vi "User32dllAPI.EnumWindows.vi"(8 "error in (no error)":errorcluster, 10 "Pattern":string, 11 "hWnd in (NULL)":i32) -> (0 "error out":errorcluster, 1 "ClassName":string[](array[string]), 2 "WindowName":string[](array[string]), 3 "hWnd out":i32)   [LabVIEW 2016]
uses:
  <vilib>/Utility/importsl/GetValueByPointer/datatype.ctl
  <vilib>/Utility/importsl/GetValueByPointer/GetValueByPointer.xnode
  User32WinApi.dll
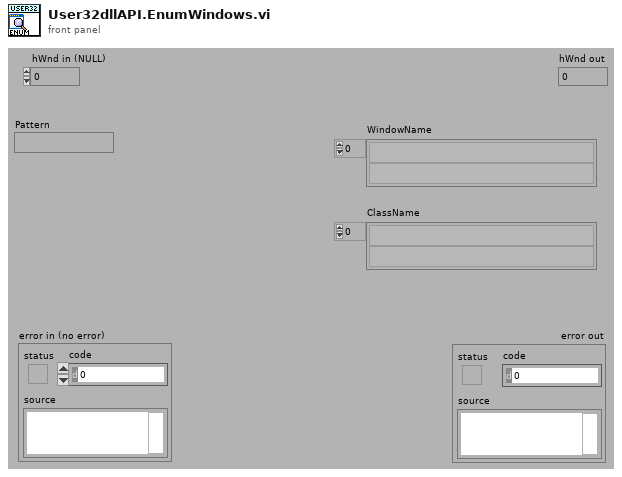
[diagram p1: front panel]
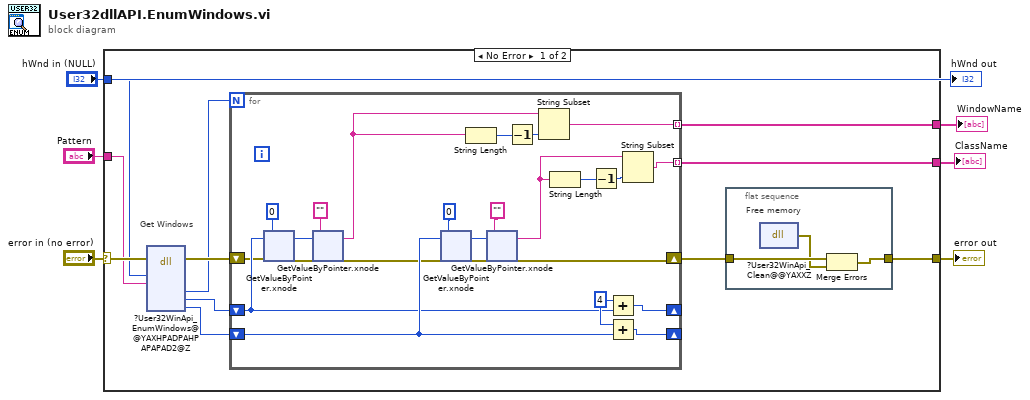
[diagram p0: block diagram]
diagram:
  n1 = case shown="No Error" "error in (no error)" {
    selector: "error in (no error)" -> [w14 w93]
    tunnel: [w8 w93] -> w5
    tunnel: [w13 _] -> w3
    tunnel: [w12 _] -> w2
    tunnel: "Pattern" -> [w11 _]
    tunnel: "hWnd in (NULL)" -> [w10 _]
    frame No Error {
      # "Get Windows"
      n2 = dll-call lib="D:/maszup/svn/LineTraceSystem/SOFTWARE/sources/Tools/Windows/User32WinApi.dll" fn="?User32WinApi_EnumWindows@@YAXHPADPAHPAPAPAD2@Z"(error in=w14, "hWnd"=w10, "cPattern"=w11) -> (error out=w17:errorcluster, "nMaxSize"=w15:i32, "winName"=w16:i64, "winClass"=w7:i64)  [unwired: 8 in, 1 out]
      n3 = for {
        N: w15 -> [_]
        shift-right: [w42] -> _
        shift-left: w16 -> [w32]
        shift-right: [w23] -> w9
        shift-left: w17 -> [w29]
        shift-right: [w43] -> _
        shift-left: w7 -> [w35]
        tunnel: [w37] -> w12 mode=indexing
        tunnel: [w36] -> w13 mode=indexing
        w44 = i64 4 ("x")
        n4 = xnode "GetValueByPointer.xnode"("Pointer"=w32, "InputType"=i64 0, "ErrorIn"=w29) -> ("Output"=w31:i64, "ErrorOut"=w30:errorcluster)  [unwired: 1 in]
        n5 = xnode "GetValueByPointer.xnode"("Pointer"=w31, "InputType"="", "ErrorIn"=w30) -> ("Output"=w21:string, "ErrorOut"=w24:errorcluster)  [unwired: 1 in]
        n6 = xnode "GetValueByPointer.xnode"("Pointer"=w35, "InputType"=i64 0, "ErrorIn"=w24) -> ("Output"=w28:i64, "ErrorOut"=w27:errorcluster)  [unwired: 1 in]
        n7 = String Length(string=w21) -> (length=w41:i32)
        n8 = xnode "GetValueByPointer.xnode"("Pointer"=w28, "InputType"="", "ErrorIn"=w27) -> ("Output"=w22:string, "ErrorOut"=w23:errorcluster)  [unwired: 1 in]
        n9 = Decrement(x=w41) -> (x-1=w40:i32)
        n10 = String Subset(string=w21, length (rest)=w40) -> (substring=w37:string)  [unwired: 1 in]
        n11 = String Length(string=w22) -> (length=w38:i32)
        n12 = Decrement(x=w38) -> (x-1=w39:i32)
        n13 = Add(x=w44, y=w32) -> (x+y=w42:i64)
        n14 = Add(x=w44, y=w35) -> (x+y=w43:i64)
        n15 = String Subset(string=w22, length (rest)=w39) -> (substring=w36:string)  [unwired: 1 in]
      }
      n16 = flat-sequence {
        tunnel: w9 -> [w20]
        tunnel: [w18] -> w8
        frame #0 {
          # "Free memory"
          n17 = dll-call lib="D:/maszup/svn/LineTraceSystem/SOFTWARE/sources/Tools/Windows/User32WinApi.dll" fn="?User32WinApi_Clean@@YAXXZ"() -> (error out=w19:errorcluster)  [unwired: 4 in, 1 out]
          n18 = Merge Errors(w20, w19) -> (w18:errorcluster)
        }
      }
    }
    frame Error {
    }
  }
  "error out" <- w5
  "ClassName" <- w3
  "WindowName" <- w2
  "hWnd out" <- "hWnd in (NULL)"
